vi "MALT Set Rapidly.vi"() -> ()   [LabVIEW 2018]
doc: "Use this template to build a user interface event handler design pattern. Use this pattern for dialog boxes and other user interfaces. You also can create and execute user-defined events that the VI can handle the same way as user interface events."
uses:
  <instrlib>/AltonTech MALT/AltonTech MALT200817.lvlib
panel:
  in  "Port":i32=4
  in  "Address":i32=3
  out "Cycle":i32
  in  "stop":bool
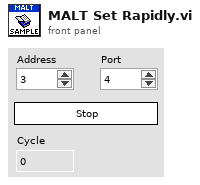
[diagram p1: front panel]
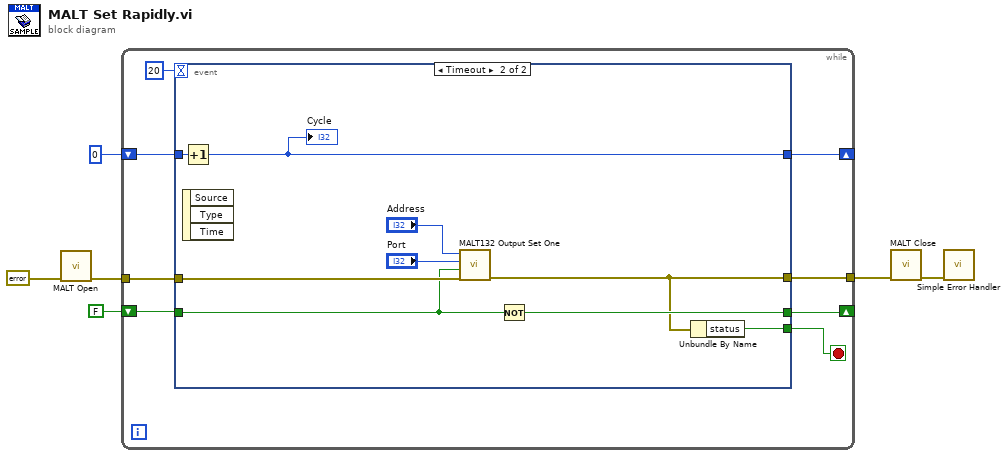
[diagram p0: block diagram]
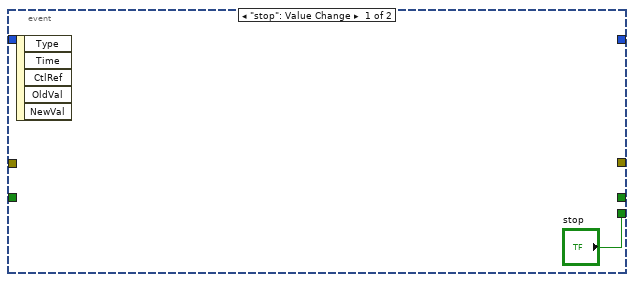
[diagram p2: hidden frame]
diagram:
  n1 = call <instrlib>:"MALT Open.vi"("error in"=errorcluster {"status"=FALSE, "code"=0, "source"=""}) -> ("error out"=w4:errorcluster)  [unwired: 10 in]
  n2 = while {
    shift-right: [w12] -> _
    shift-left: FALSE -> [w11]
    tunnel: w4 -> [w10]
    shift-right: [w8] -> _
    shift-left: 0 -> [w9]
    tunnel: [w7] -> w2
    stop <- w14 stop-if-true
    n3 = event shown="[1] Timeout" {
      selector: _ -> [_ _]
      dyn-events: _ -> [_ _]
      timeout: 20 -> [_ _]
      tunnel: ["stop" w17] -> w14
      tunnel: w11 -> [_ w16]
      tunnel: [_ w22] -> w12
      tunnel: w10 -> [_ w21]
      tunnel: w9 -> [_ w24]
      tunnel: [_ w23] -> w8
      tunnel: [_ w20] -> w7
      event "stop": Value Change {
        n4 = event-data() -> ()  [unwired: 1 in, 5 out]
      }
      event Timeout {
        n5 = Increment(x=w24) -> (x+1=w23:i32)
        "Cycle" <- w23
        n6 = event-data() -> ()  [unwired: 1 in, 3 out]
        n7 = call <instrlib>:"MALT132 Output Set One.vi"("error in"=w21, "State"=w16, "Relay Num"="Port", "Address"="Address") -> ("error out"=w20:errorcluster)  [unwired: 7 in]
        n8 = Not(x=w16) -> (.not. x?=w22:bool)
        n9 = Unbundle By Name(w20) -> ("status"=w17:bool)
      }
    }
  }
  n10 = call <instrlib>:"MALT Close.vi"("error in"=w2) -> ("error out"=w1:errorcluster)  [unwired: 10 in]
  n11 = call <vilib>:"Simple Error Handler.vi"("error in (no error)"=w1) -> ()  [unwired: 4 in, 5 out]
